vi "Acquire Class Details.vi"(8 "error in":errorcluster, 11 "Class Path":path) -> (0 "error out":errorcluster, 1 "Member VI info":T2[](array[typedef]), 2 "Hierarchy Array":T1[](array[typedef]), 3 "Class Info":T1, 5 "Is Interface":bool)   [LabVIEW 2020, in "ClassLoader.lvlib"]
doc: "Obtain class data using VI server."
uses:
  ClassLoader.lvlib
  <vilib>/Utility/Data Type/Member VI Info.ctl
  Ctl/Ctl_Class Info.ctl
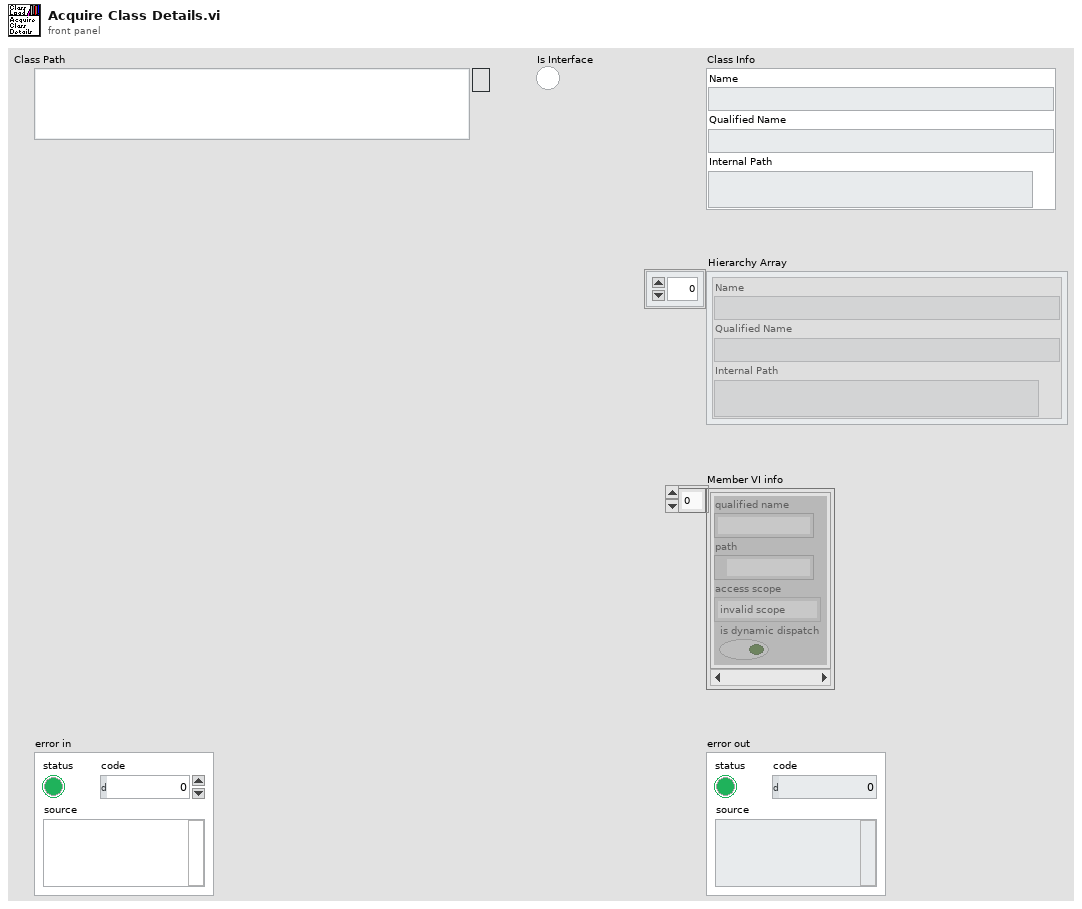
[diagram p1: front panel]
types:
  T1 = typedef "ClassLoader.lvlib/Ctl_Class Info.ctl" = cluster{"Name":string, "Qualified Name":string, "Internal Path":string}
  T2 = typedef "Member VI Info.ctl" = cluster{"qualified name":string, "path":path, "access scope":enum32{"invalid scope", "public", "private", "protected", "community"}, "is dynamic dispatch":bool}
  T3 = cluster{"Static Member VIs":refnum<vi>[], "is dynamic dispatch":bool}
  T4 = cluster{"Dynamic Member VIs":refnum<vi>[], "is dynamic dispatch":bool}
  T5 = cluster{"Dynamic Member VIs":refnum<vi>[], "is dynamic dispatch":bool}[]
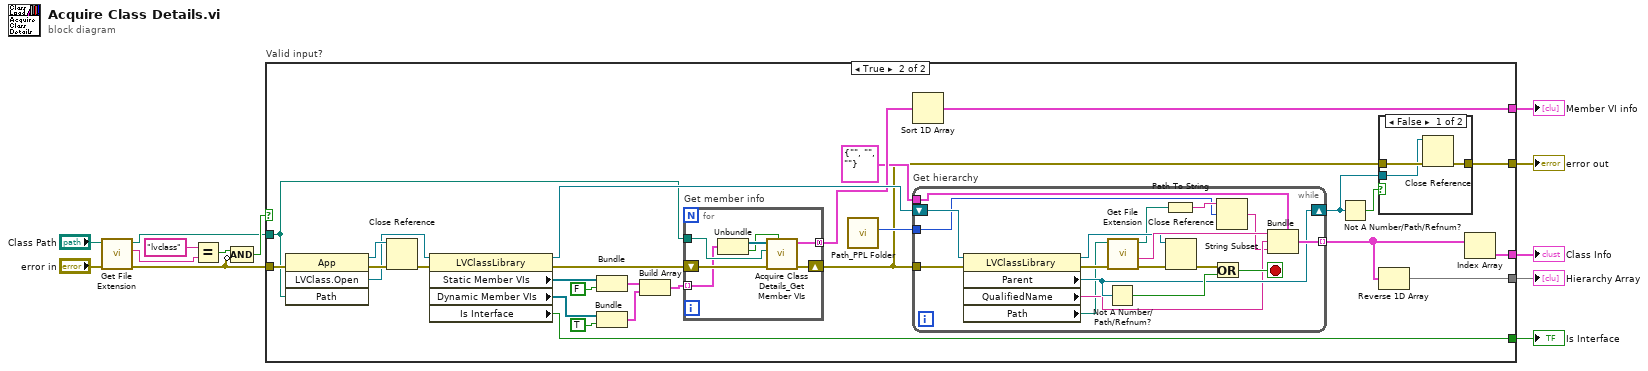
[diagram p0: block diagram]
diagram:
  n1 = call <vilib>:"Get File Extension.vi"("error in (no error)"="error in", "file"="Class Path") -> ("error out"=w7:errorcluster, "lowercase file extension"=w13:string, "dup file"=w6:path)  [unwired: 5 in, 2 out]
  n2 = Equal?(x="lvclass", y=w13) -> (x = y?=w11:bool)
  n3 = Compound Arithmetic op=AND(w11, invert w7) -> (w9:bool)
  n4 = case "Valid input?" shown="True" w9 {
    tunnel: [w14 w38] -> w8
    tunnel: w7 -> [w14 w39]
    tunnel: w6 -> [_ w24]
    tunnel: [_ w37] -> w5
    tunnel: [_ w28] -> w4
    tunnel: [_ w30] -> w3
    tunnel: [_ w26] -> w2
    frame False {
    }
    frame True {
      n5 = invoke class="App" method="LVClass.Open"(error in=w39, "Path"=w24) -> (reference out=w40:refnum<vi>, error out=w41:errorcluster, "LVClass.Open"=w34:refnum<vi>)  [unwired: 2 in, 1 out]
      n6 = Close Reference(reference=w40, error in (no error)=w41) -> (error out=w32:errorcluster)
      n7 = property class="LVClassLibrary"(reference=w34, error in=w32) -> (reference out=w33:refnum<vi>, error out=w31:errorcluster, "Static Member VIs"=w22:refnum<vi>[], "Dynamic Member VIs"=w19:refnum<vi>[], "Is Interface"=w30:bool)
      n8 = Bundle("Static Member VIs"=w22, "is dynamic dispatch"=FALSE) -> (w18:T3)  [unwired: 1 in]
      n9 = Bundle("Dynamic Member VIs"=w19, "is dynamic dispatch"=TRUE) -> (w17:T4)  [unwired: 1 in]
      n10 = Build Array(w18, w17) -> (w16:T5)
      n11 = for "Get member info" {
        tunnel: [w46] -> w29 mode=concatenating
        tunnel: w24 -> [w45]
        shift-right: [w47] -> w15
        shift-left: w31 -> [w48]
        tunnel: w16 -> [w44] mode=indexing
        n12 = Unbundle(w44) -> ("Dynamic Member VIs"=w43:refnum<vi>[], "is dynamic dispatch"=w42:bool)
        n13 = call "Acquire Class Details_Get Member VIs.vi"("Dynamic dispatch?"=w42, "error in (no error)"=w48, "Class Path"=w45, "Member VIs (auto closed)"=w43) -> ("error out"=w47:errorcluster, "Member Array"=w46:T2[])  [unwired: 6 in]
      }
      n14 = call "Path_PPL Folder.vi"() -> ("Path Length"=w23:i32)  [unwired: 10 in, 1 out]
      n15 = Sort 1D Array(array=w29) -> (sorted array=w28:T2[])
      n16 = while "Get hierarchy" {
        shift-right: [w62] -> w36
        shift-left: w33 -> [w63]
        tunnel: [w69] -> w27 mode=indexing
        tunnel: w15 -> [w66]
        tunnel: T1 {"Name"="", "Qualified Name"="", "Internal Path"=""} ("Class Info") -> [w57]
        tunnel: w23 -> [w55]
        stop <- w67 stop-if-true
        n17 = property class="LVClassLibrary"(reference=w63, error in=w66) -> (reference out=w61:refnum<vi>, error out=w60:errorcluster, "Parent"=w62:refnum<vi>, "QualifiedName"=w59:string, "Path"=w58:path)
        n18 = Not A Number/Path/Refnum?(number/path/refnum=w62) -> (NaN/Path/Refnum?=w70:bool)
        n19 = call <vilib>:"Get File Extension.vi"("error in (no error)"=w60, "file"=w58) -> ("error out"=w65:errorcluster, "filename without extension"=w64:string, "dup file"=w54:path)  [unwired: 5 in, 2 out]
        n20 = Path To String(path=w54) -> (string=w56:string)
        n21 = Close Reference(reference=w61, error in (no error)=w65) -> (error out=w68:errorcluster)
        n22 = Or(x=w68, y=w70) -> (x .or. y?=w67:bool)
        n23 = String Subset(string=w56, offset (0)=w55) -> (substring=w53:string)  [unwired: 1 in]
        n24 = Bundle(cluster=w57, "Name"=w64, "Qualified Name"=w59, "Internal Path"=w53) -> (w69:T1)
      }
      n25 = Not A Number/Path/Refnum?(number/path/refnum=w36) -> (NaN/Path/Refnum?=w35:bool)
      n26 = case shown="False" w35 {
        tunnel: w15 -> [w51 w52]
        tunnel: [w50 w52] -> w38
        tunnel: w36 -> [w49 _]
        frame False {
          n27 = Close Reference(reference=w49, error in (no error)=w51) -> (error out=w50:errorcluster)
        }
        frame True {
        }
      }
      n28 = Reverse 1D Array(array=w27) -> (reversed array=w37:T1[])
      n29 = Index Array(array=w27) -> (element=w26:T1)  [unwired: 1 in]
    }
  }
  "error out" <- w8
  "Member VI info" <- w4
  "Hierarchy Array" <- w5
  "Is Interface" <- w3
  "Class Info" <- w2
